vi "CANOpen_Read SDOs Data.vi"(8 "error in":errorcluster, 11 "SDO Asynch":T1 {"HW Dyn Read"."Resp Chan."."Chan Refs" format="%.0x"; "HW Dyn Read"."Req Chan."."Chan Refs" format="%.0x"; "HW Dyn Write"."Resp Chan."."Chan Refs" format="%.0x"; "HW Dyn Write"."Req Chan."."Chan Refs" format="%.0x"; "List SDO"."Resp Chan."."Chan Refs" format="%.0x"; "List SDO"."Req Chan."."Chan Refs" format="%.0x"}) -> (0 "error out":errorcluster, 3 "SDO Asynch out":T1 {"HW Dyn Read"."Resp Chan."."Chan Refs" format="%.0x"; "HW Dyn Read"."Req Chan."."Chan Refs" format="%.0x"; "HW Dyn Write"."Resp Chan."."Chan Refs" format="%.0x"; "HW Dyn Write"."Req Chan."."Chan Refs" format="%.0x"; "List SDO"."Resp Chan."."Chan Refs" format="%.0x"; "List SDO"."Req Chan."."Chan Refs" format="%.0x"})   [LabVIEW 2013, in "CANOpen Addon Custom Device.lvlib"]
uses:
  CANOpen Addon Custom Device.lvlib
  CANOpen_VS SDOs Data Refs.ctl
  <vilib>/NI Veristand/Custom Device API/Data Reference.ctl
  Async VIs/CANOpen_Main/SubVIs/CanOpen_SDO Dynamic queue.ctl
  Shared Code/CANOpen_SDO queue W data.ctl
  Shared Code/CANOpen_SDO queue mode.ctl
  Shared Code/CANOpen_PDO Data Type in queue.ctl
  <vilib>/NI Veristand/Custom Device API/NI VeriStand - Set Channel Value by Data Reference.vi
  <vilib>/NI Veristand/Custom Device API/NI VeriStand - Get Channel Value by Data Reference.vi
  CANOpen_SDO Update status channels Dyn Read.vi
  CANOpen_SDO Update status channels Dyn Write.vi
  <vilib>/NI Veristand/Custom Device API/Global Data Refs.vi
  <vilib>/NI Veristand/Custom Device API/Custom Device API.lvlib
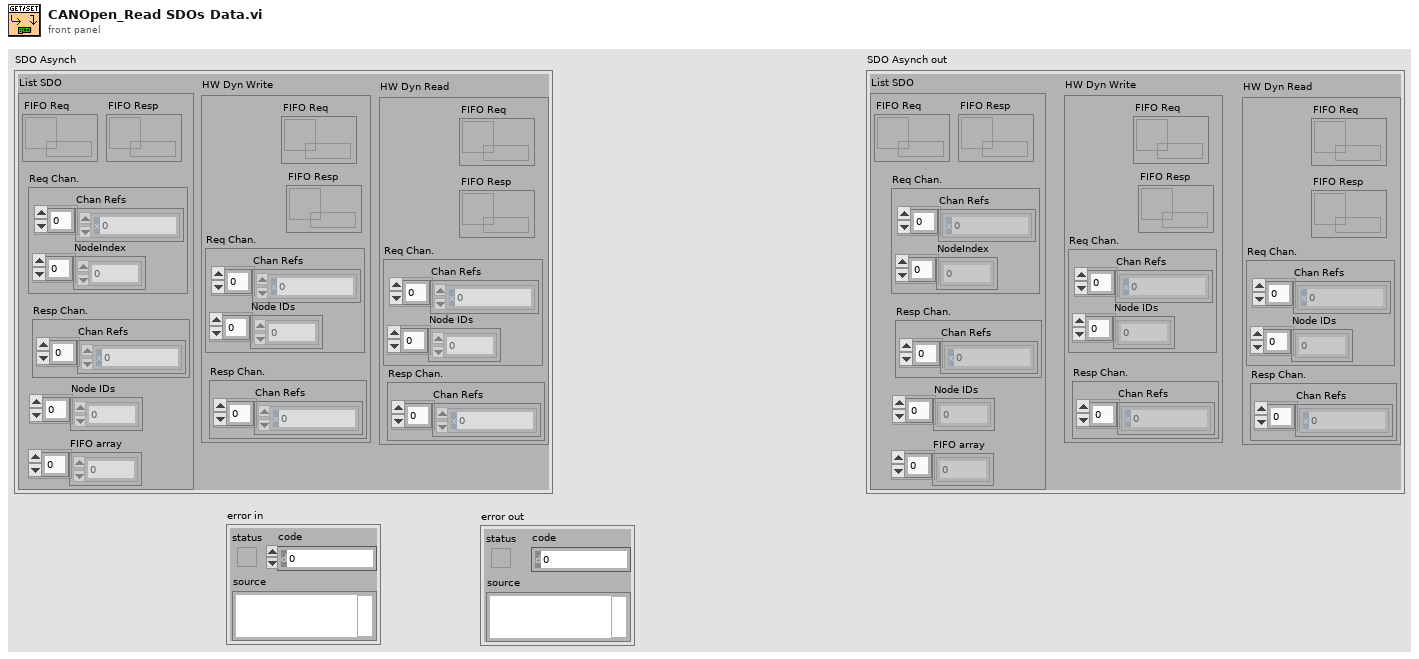
[diagram p1: front panel]
types:
  T1 = typedef "CANOpen Addon Custom Device.lvlib/CANOpen_VS SDOs Data Refs.ctl" = cluster{"List SDO":cluster{"FIFO Req":refnum<k33>, "Req Chan.":cluster{"Chan Refs":T2[], "NodeIndex":dbl[]}, "FIFO Resp":refnum<k33>, "Resp Chan.":cluster{"Chan Refs":T2[]}, "Node IDs":u8[], "FIFO array":dbl[]}, "HW Dyn Write":cluster{"FIFO Req":refnum<k33>, "FIFO Resp":refnum<k33>, "Req Chan.":cluster{"Chan Refs":T2[], "Node IDs":u8[]}, "Resp Chan.":cluster{"Chan Refs":T2[]}}, "HW Dyn Read":cluster{"FIFO Req":refnum<k33>, "FIFO Resp":refnum<k33>, "Req Chan.":cluster{"Chan Refs":T2[], "Node IDs":u8[]}, "Resp Chan.":cluster{"Chan Refs":T2[]}}}
  T2 = typedef "Custom Device API.lvlib/Data Reference.ctl" = i32
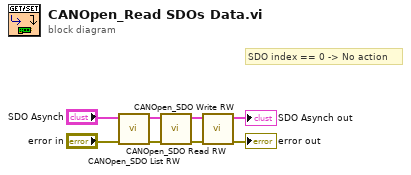
[diagram p0: block diagram]
diagram:
  # "SDO index == 0 -> No action"
  n1 = call "CANOpen_SDO List RW.vi"("error in (no error)"="error in", "SDO Asynch in"="SDO Asynch") -> ("error out"=w7:errorcluster, "SDO Asynch out"=w2:T1)  [unwired: 8 in]
  n2 = call "CANOpen_SDO Read RW.vi"("error in"=w7, "SDO Asynch in"=w2) -> ("error out"=w6:errorcluster, "SDO Asynch out"=w1:T1)  [unwired: 8 in]
  n3 = call "CANOpen_SDO Write RW.vi"("error in"=w6, "SDO Asynch in"=w1) -> ("error out"=→"error out":errorcluster, "SDO Asynch out"=→"SDO Asynch out":T1)  [unwired: 8 in]
